vi "draw - 4 corner circle.vi"(8 "4corners":T1={"z (-pi/2)"=-1.0311345636926572+0.5736824521422934i, "z(inf)"=-0.5200164984937075+1.0975277942502903i, "z (pi/2)"=-1.0311345636926572+0.5736824521422934i, "z center"=-0.5136528600391839+0.580046090596817i, "z(0)"=-0.5200164984937075+1.0975277942502903i, "radius"=-1.0311345636926572}) -> (0 "line two":cluster{dbl[], dbl[]}, 1 "line one":cluster{dbl[], dbl[]}, 2 "circle":cluster{dbl[], dbl[]})   [LabVIEW 2018]
uses:
  circle corners.ctl
  generate linear region.vi
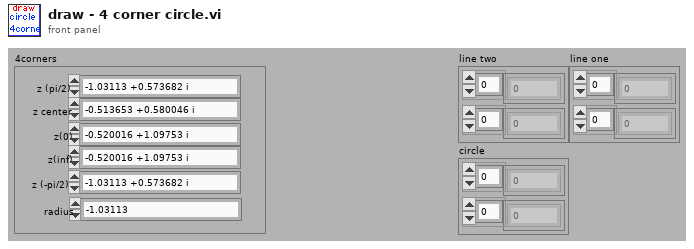
[diagram p1: front panel]
types:
  T1 = typedef "circle corners.ctl" = cluster{"z (-pi/2)":cdb, "z(inf)":cdb, "z (pi/2)":cdb, "z center":cdb, "z(0)":cdb, "radius":dbl}
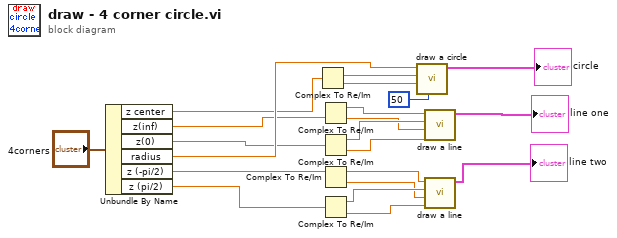
[diagram p0: block diagram]
diagram:
  n1 = Unbundle By Name("4corners") -> ("z center"=w6:cdb, "z(inf)"=w8:cdb, "z(0)"=w7:cdb, "radius"=w15:dbl, "z (-pi/2)"=w10:cdb, "z (pi/2)"=w9:cdb)
  n2 = Complex To Re/Im(x + iy=w6) -> (x=w16:dbl, y=w17:dbl)
  n3 = Complex To Re/Im(x + iy=w8) -> (x=w21:dbl, y=w19:dbl)
  n4 = Complex To Re/Im(x + iy=w7) -> (x=w20:dbl, y=w18:dbl)
  n5 = Complex To Re/Im(x + iy=w10) -> (x=w14:dbl, y=w12:dbl)
  n6 = Complex To Re/Im(x + iy=w9) -> (x=w13:dbl, y=w11:dbl)
  n7 = call "draw a circle.vi"("number of points"=50, "center Y"=w17, "center x"=w16, "radius"=w15) -> ("output cluster"=→"circle":cluster{dbl[], dbl[]})  [unwired: 7 in]
  n8 = call "draw a line.vi"("y1"=w18, "y0"=w19, "x1"=w20, "x0"=w21) -> ("output cluster"=→"line one":cluster{dbl[], dbl[]})  [unwired: 7 in]
  n9 = call "draw a line.vi"("y1"=w11, "y0"=w12, "x1"=w13, "x0"=w14) -> ("output cluster"=→"line two":cluster{dbl[], dbl[]})  [unwired: 7 in]
